vi "Init.vi"(8 "error in (no error)":errorcluster, 10 "ID":string, 11 "DC Motor in":refnum<class "DC Motor.lvclass">) -> (0 "error out":errorcluster, 3 "DC Motor out":refnum<class "DC Motor.lvclass">)   [LabVIEW 2021, in "DC Motor.lvclass"]
uses:
  DC Motor.lvclass
  DC Motor.lvclass/DC Motor.ctl
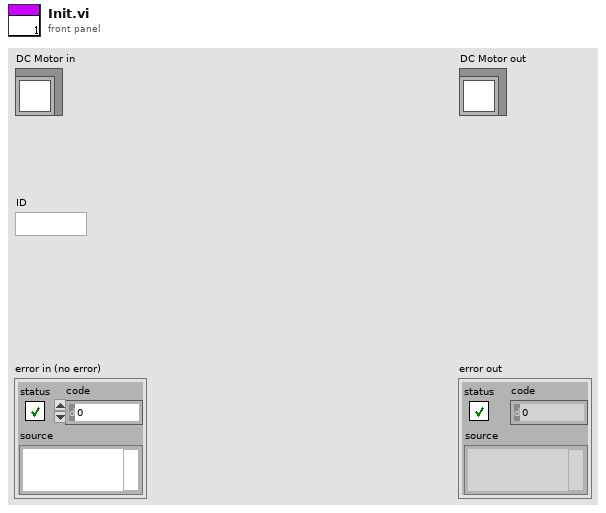
[diagram p1: front panel]
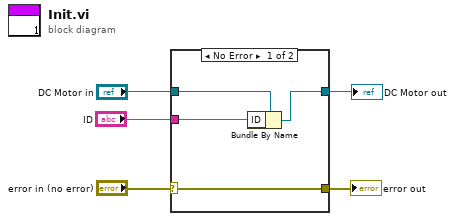
[diagram p0: block diagram]
diagram:
  n1 = case shown="No Error" "error in (no error)" {
    selector: "error in (no error)" -> [w9 w11]
    tunnel: [w9 w11] -> w4
    tunnel: [w7 w10] -> w3
    tunnel: "DC Motor in" -> [w8 w10]
    tunnel: "ID" -> [w6 _]
    frame No Error {
      n2 = Bundle By Name(cluster=w8, "ID"=w6) -> (w7:refnum<class "DC Motor.lvclass">)
    }
    frame Error {
    }
  }
  "error out" <- w4
  "DC Motor out" <- w3
